vi "dialog.vi"(4 "Sequence Context":T1) -> (0 "error out":errorcluster, 1 "Test Data":T2 {"Numeric Measurement" format="%.2f"})   [LabVIEW 2013]
uses:
  Demo/LabVIEW/SupportVIs.llb/LabVIEW Test - Test Data.ctl
  <vilib>/addons/TestStand/_TSLegacy.llb/LabVIEW Test - Sequence Context.ctl
  <vilib>/addons/TestStand/_TSUtility.llb/TestStand - Start Modal Dialog (Sequence Context).vi
  <vilib>/addons/TestStand/_TSUtility.llb/TestStand - End Modal Dialog (Sequence Context).vi
panel:
  in  "Boolean":bool
  # "This VI is an example of a dialog box that is modal to the TestStand\nmain application window. See the diagram of this VI for information\non how to create such a VI."
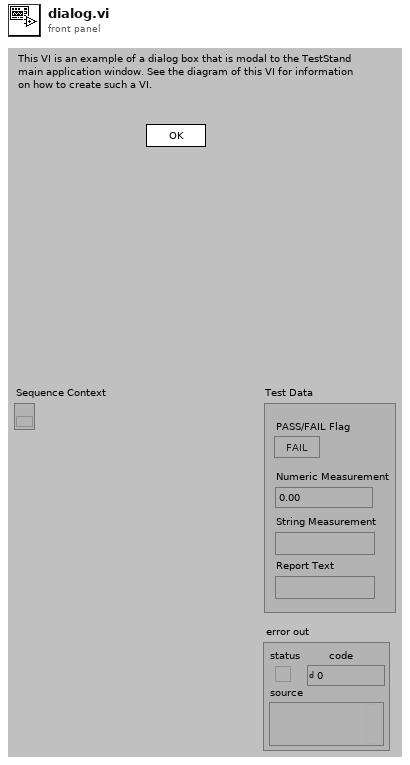
[diagram p1: front panel]
types:
  T1 = typedef "LabVIEW Test - Sequence Context.ctl" = refnum<k7>
  T2 = typedef "LabVIEW Test - Test Data.ctl" = cluster{"PASS/FAIL Flag":bool, "Numeric Measurement":dbl, "String Measurement":string, "Report Text":string}
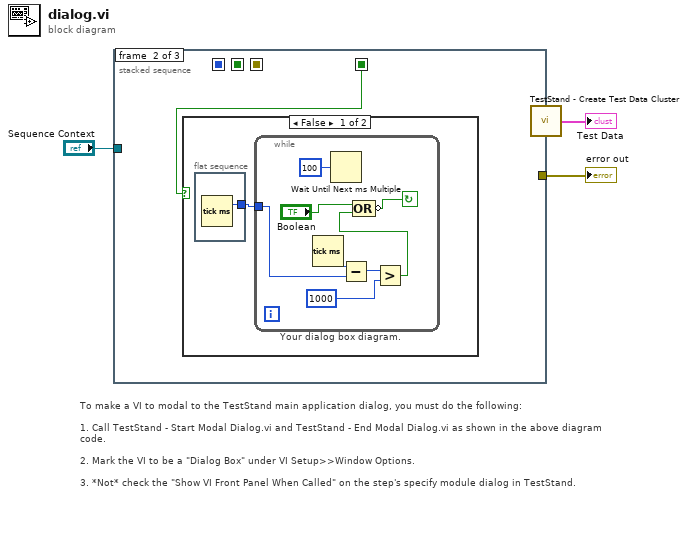
[diagram p0: block diagram]
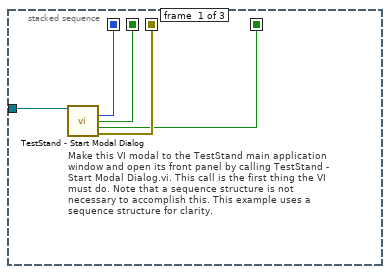
[diagram p2: hidden frame]
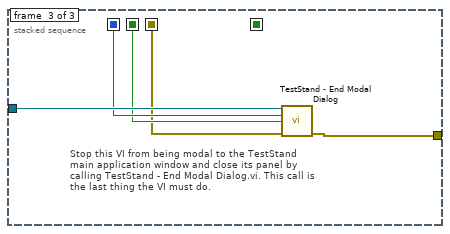
[diagram p4: hidden frame]
diagram:
  # "To make a VI to modal to the TestStand main application dialog, you must do the following:\n\n1. Call TestStand - Start Modal Dialog.vi and TestStand - End Modal Dialog.vi as shown in the above diagram code.\n\n2. Mark the VI to be a \"Dialog Box\" under VI Setup>>Window Options.\n\n3. *Not* check the \"Show VI Front Panel When Called\" on the step's specify module dialog in TestStand."
  n1 = stacked-sequence {
    seq-local: [w5 _ _] -> [_ _ w21]
    seq-local: [w7 _ _] -> [_ _ w23]
    seq-local: [w6 _ _] -> [_ _ w22]
    seq-local: [w4 _ _] -> [_ w9 _]
    tunnel: "Sequence Context" -> [w8 _ w24]
    tunnel: [_ _ w20] -> w1
    frame #0 {
      # "Make this VI modal to the TestStand main application\nwindow and open its front panel by calling TestStand -\nStart Modal Dialog.vi. This call is the first thing the VI\nmust do. Note that a sequence structure is not\nnecessary to accomplish this. This example uses a\nsequence structure for clarity."
      n2 = call-poly <vilib>:"TestStand - Start Modal Dialog.vi"("Sequence Context In"=w8) -> ("Modal ID"=w7:i32, "VI Originally Open"=w6:bool, "Should Abort"=w4:bool, "error out"=w5:errorcluster)  [unwired: 10 in, 1 out]
    }
    frame #1 {
      n3 = case shown="False" w9 {
        frame False {
          # "Your dialog box diagram."
          n4 = flat-sequence {
            tunnel: [w11] -> w10
            frame #0 {
              n5 = Tick Count (ms)() -> (millisecond timer value=w11:u32)
            }
          }
          n6 = while {
            tunnel: w10 -> [w15]
            stop <- w12 continue-if-true
            n7 = Tick Count (ms)() -> (millisecond timer value=w17:u32)
            n8 = Wait Until Next ms Multiple(millisecond multiple=u32 100) -> ()  [unwired: 1 out]
            n9 = Subtract(x=w17, y=w15) -> (x-y=w18:u32)
            n10 = Greater?(x=w18, y=u32 1000) -> (0:w13:bool)
            n11 = Compound Arithmetic op=OR("Boolean", w13) -> (invert w12:bool)
          }
        }
        frame True {
        }
      }
    }
    frame #2 {
      # "Stop this VI from being modal to the TestStand main application window and close its panel by calling TestStand - End Modal Dialog.vi. This call is the last thing the VI must do."
      n12 = call-poly <vilib>:"TestStand - End Modal Dialog.vi"("Sequence Context In"=w24, "Modal ID"=w23, "VI Originally Open"=w22, "error in (no error)"=w21) -> ("error out"=w20:errorcluster)  [unwired: 11 in]
    }
  }
  "error out" <- w1
  n13 = call "TestStand - Create Test Data Cluster.vi"() -> ("Test Data"=→"Test Data":T2)  [unwired: 4 in]
